vi "Configure Timebase (Reference).vi"(0 "VISA resource name":refnum<visa-resource-name>, 5 "Time Reference Location (0.5)":dbl=0.5, 11 "error in (no error)":errorcluster) -> (4 "VISA resource name out":refnum<visa-resource-name>, 15 "error out":errorcluster)   [LabVIEW 2017, in "Agilent 2000 3000 X-Series.lvlib"]
doc: "Configure the time reference location at a percent of the graticule width. \n\n<b>Note:</b>\n - This VI is only applicable for 3000T, 4000, 6000 X-Series.\n - You should call <b>Configure Timebase (Basic)</b> and set the timebase reference to custom before call this VI."
uses:
  Agilent 2000 3000 X-Series.lvlib
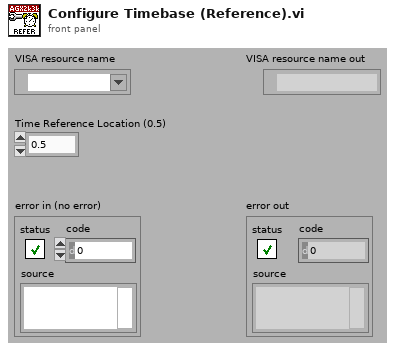
[diagram p1: front panel]
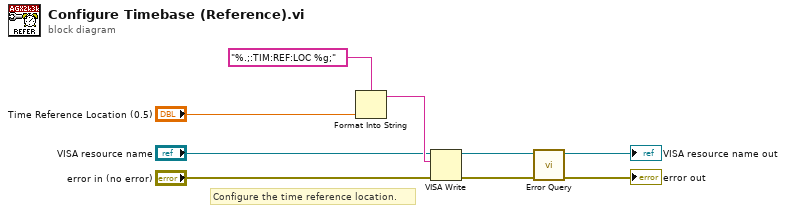
[diagram p0: block diagram]
diagram:
  # "Configure the time reference location."
  n1 = Format Into String(format string="%.;:TIM:REF:LOC %g;", "Time Reference Location (0.5)") -> (resulting string=w7:string)  [unwired: 2 in, 1 out]
  n2 = VISA Write(VISA resource name="VISA resource name", write buffer=w7, error in (no error)="error in (no error)") -> (VISA resource name out=w4:refnum<visa-resource-name>, error out=w3:errorcluster)  [unwired: 1 out]
  n3 = call "Error Query.vi"("error in (no error)"=w3, "VISA resource name"=w4) -> ("error out"=→"error out":errorcluster, "VISA resource name out"=→"VISA resource name out":refnum<visa-resource-name>)  [unwired: 6 in, 2 out]
